vi "createPubDataEvents.vi"(8 "error in (no error)":errorcluster, 11 "DataListenerThisComponent in":refnum<class "DataListenerThisComponent.lvclass">) -> (0 "error out":errorcluster, 3 "DataListenerThisComponent out":refnum<class "DataListenerThisComponent.lvclass">)   [LabVIEW 2015]
uses:
  Typedefs/StateValue.ctl
  Typedefs/EXATypedefs.lvlib
  Typedefs/CommandValue.ctl
  Typedefs/RejectedCommand.ctl
  ComponentTemplateCore_UserEvents/ComponentModel/ComponentModel/Typedefs/ComponentStateValues.ctl
  DataListenerThisComponent.lvclass
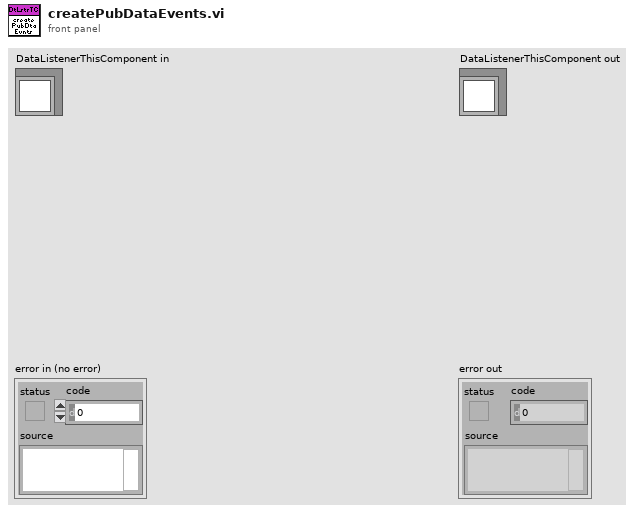
[diagram p1: front panel]
types:
  T1 = typedef "ComponentStateValues.ctl" = enum16{"Off", "Standby", "Enabled", "Disabled", "Fault"}
  T2 = typedef "EXATypedefs.lvlib/RejectedCommand.ctl" = cluster{"CommandValue":T3, "StateValue":T4, "Time Stamp":timestamp}
  T3 = typedef "EXATypedefs.lvlib/CommandValue.ctl" = enum16{"ClearError", "Disable", "Enable", "Exit", "GoToStandby", "OnHeartbeat", "OnIncomingMessagingError", "OnInterrupt", "Start"}
  T4 = typedef "EXATypedefs.lvlib/StateValue.ctl" = enum16{"DisabledState", "EnabledState", "FaultState", "OffState", "StandbyState"}
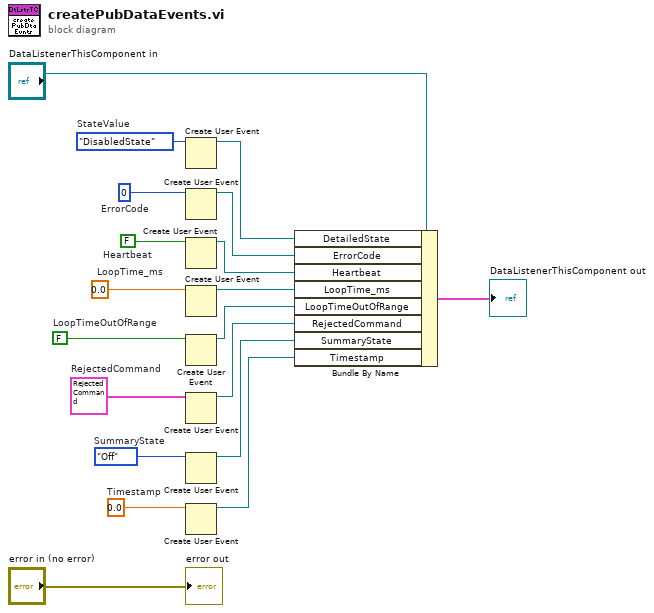
[diagram p0: block diagram]
diagram:
  w12 = 0.0  # Timestamp
  w13 = ComponentStateValues."Off"  # SummaryState
  w14 = T2 {"CommandValue"=enum."ClearError", "StateValue"=enum."DisabledState", "Time Stamp"=timestamp(0 s since 1904-01-01)}  # RejectedCommand
  w15 = FALSE  # LoopTimeOutOfRange
  w16 = 0.0  # LoopTime_ms
  w17 = FALSE  # Heartbeat
  w18 = 0  # ErrorCode
  w19 = StateValue."DisabledState"  # StateValue
  n1 = Create User Event(user event datatype=w19) -> (user event=w11:refnum<user-event>)  [unwired: 1 in, 1 out]
  n2 = Create User Event(user event datatype=w18) -> (user event=w8:refnum<user-event>)  [unwired: 1 in, 1 out]
  n3 = Create User Event(user event datatype=w17) -> (user event=w7:refnum<user-event>)  [unwired: 1 in, 1 out]
  n4 = Create User Event(user event datatype=w16) -> (user event=w6:refnum<user-event>)  [unwired: 1 in, 1 out]
  n5 = Create User Event(user event datatype=w15) -> (user event=w5:refnum<user-event>)  [unwired: 1 in, 1 out]
  n6 = Create User Event(user event datatype=w14) -> (user event=w4:refnum<user-event>)  [unwired: 1 in, 1 out]
  n7 = Create User Event(user event datatype=w13) -> (user event=w3:refnum<user-event>)  [unwired: 1 in, 1 out]
  n8 = Create User Event(user event datatype=w12) -> (user event=w2:refnum<user-event>)  [unwired: 1 in, 1 out]
  n9 = Bundle By Name(cluster="DataListenerThisComponent in", "DetailedState"=w11, "ErrorCode"=w8, "Heartbeat"=w7, "LoopTime_ms"=w6, "LoopTimeOutOfRange"=w5, "RejectedCommand"=w4, "SummaryState"=w3, "Timestamp"=w2) -> (→"DataListenerThisComponent out":cluster{})
  "error out" <- "error in (no error)"
